vi "Get Attribute.Instrument.vi"(8 "error in (no error)":errorcluster, 11 "SMO":refnum<class "SMO.lvclass">) -> (0 "error out":errorcluster, 2 "Attribute.Debug":refnum<class "Attribute.Instrument.lvclass">, 3 "SMO out":refnum<class "SMO.lvclass">)   [LabVIEW 2019, in "Instrument Attributes.lvlib" / "SMO.Mediator.lvclass"]
uses:
  SMO.Mediator.lvclass
  <vilib>/JKI/JKI SMO/SMO/SMO.lvclass
  Attribute.Instrument/Attribute.Instrument.lvclass
  C:/Program Files (x86)/National Instruments/LabVIEW 2019/vi.lib/JKI/JKI SMO/Support/Attribute/Attribute.lvclass
  <vilib>/JKI/JKI SMO/Support/Attribute/Attribute.lvclass/Attribute.ctl
  <vilib>/Utility/LVClass/Get LV Class Name.vi
  <vilib>/JKI/JKI SMO/Support/Attribute/Attribute.lvclass
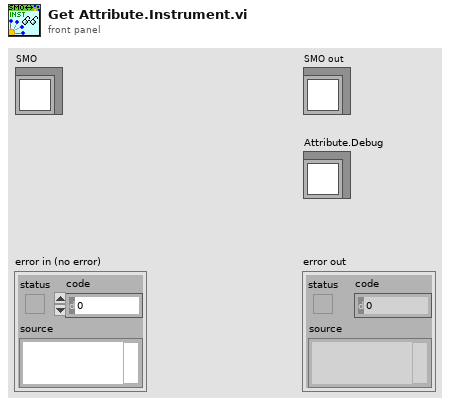
[diagram p1: front panel]
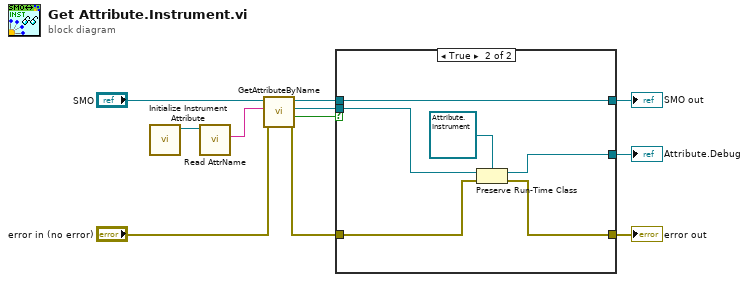
[diagram p0: block diagram]
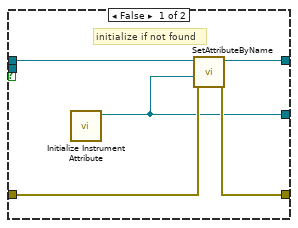
[diagram p2: hidden frame]
diagram:
  n1 = call "Initialize Instrument Attribute.vi"() -> ("Attribute.Instrument out"=w4:refnum<class "Attribute.Instrument.lvclass">)  [unwired: 11 in]
  n2 = call <vilib>:"Read AttrName.vi"("Attribute in"=w4) -> ("Attribute Name"=w3:string)  [unwired: 8 in, 2 out]
  n3 = call <vilib>:"GetAttributeByName.vi"("error in (no error)"="error in (no error)", "AttrName"=w3, "SMO in"="SMO") -> ("error out"=w5:errorcluster, "found"=w8:bool, "Attribute"=w10:refnum<class "Attribute.lvclass">, "SMO out"=w2:refnum<class "SMO.lvclass">)  [unwired: 5 in]
  n4 = case shown="True" w8 {
    tunnel: w10 -> [_ w22]
    tunnel: [w12 w17] -> w9
    tunnel: [w15 w20] -> w6
    tunnel: w5 -> [w14 w19]
    tunnel: w2 -> [w16 w18]
    tunnel: [w13 w18] -> w1
    frame False {
      # "initialize if not found"
      n5 = call "Initialize Instrument Attribute.vi"() -> ("Attribute.Instrument out"=w12:refnum<class "Attribute.Instrument.lvclass">)  [unwired: 11 in]
      n6 = call <vilib>:"SetAttributeByName.vi"("error in (no error)"=w14, "Attribute"=w12, "SMO in"=w16) -> ("error out"=w15:errorcluster, "SMO out"=w13:refnum<class "SMO.lvclass">)  [unwired: 6 in, 1 out]
    }
    frame True {
      n7 = Preserve Run-Time Class(object in=w22, error in=w19, 2:refnum<class "Attribute.Instrument.lvclass"> refnum ("SMO Debug.lvlib:Attribute.Debug.lvclass")) -> (object out=w17:refnum<class "Attribute.Instrument.lvclass">, error out=w20:errorcluster)
    }
  }
  "error out" <- w6
  "Attribute.Debug" <- w9
  "SMO out" <- w1
